vi "ReCalc_V2.00.vi"(3 "Berechnen":bool, 4 "Datenspeicher":T2={"Fahrzeugdaten"="", "date/time string"="", "Rolle [Inkr/U]"=0, "Rollenumfang [m]"=0.0, "Rollenträgheit [kgm²]"=0.0, "Zündung [Imp/U]"=0.0, "Getriebe [1:]"=0.0, "Reifenumfang [m] "=0.0, "element"=0.0, "Gl. Mittelwert"=0, "Differenzenquotient"=0, "Polynom"=0, "dT [s]"=0.0, "element"=0.0, "Lufttemperatur [°C]"=0.0, "Luftfeuchtigkeit [%]"=0.0, "Luftdruck [mbar]"=0.0, [], [], "Best Polynomial Fit"=[], [], "Übersetzung ermitteln aus"=0, "[s]"=0.0, "nmin [1/min]"=0.0, "nmax [1/min]"=0.0, "n vom Gas [1/min]"=0.0, "dT ungefiltert [s]"=[], [], "Boolesch"=FALSE, "Serielle Schnittstelle"="COM4", "nKuWe/nRolle 2"=10.0}) -> ()   [LabVIEW 2014]
uses:
  <vilib>/Utility/miscctls.llb/LVPointTypeDef.ctl
  <vilib>/Utility/xml.llb/Read From XML File(string).vi
  <vilib>/Analysis/3filter.llb/IIR Filter (DBL).vi
  <vilib>/Analysis/NI_AALBase.lvlib
panel:
  in  "Legende":bool=TRUE
  out "Fahrzeugdaten":string
  out "Überlagerung":bool
  in  "Überlagern":bool
  out "Übersetzung ermitteln aus":T1(ring)
  in  "Speichern":bool
  out "Reifenumfang [m]":dbl=1.222
  out "Getriebe [1:]":dbl=5.343
  out "Zündung [Imp/U]":dbl=1.0
  out "Rollengeber [Inkr/U]":u16=200
  out "Luftdruck [mbar]":dbl=1013.0
  out "Luftfeuchtigkeit [%]":dbl=50.0
  out "Lufttemperatur [°C]":dbl=20.0
  in  "Stopp":bool
  in  "Rollenträgheit [kgm²]":dbl=0.402
  in  "Gl. Mittelwert":u8=35
  in  "Differenzenquotient":u8=12
  in  "n vom Gas [1/min]":dbl=5000.0
  out "Rollenumfang [m]":dbl=0.613 format="%.3f"
  out "Datum, Zeit":string
  out "Untersetzung aus:":dbl=2.68 format="%.2f"
  in  "Drucken":bool
  out "Pmax":string
  out "Ergebnis":string
  out "XY-Graph":cluster{dbl[], dbl[]}[](graph)
  in  "Öffnen":bool
  out "korr":dbl
  out "[s]":dbl=5.0
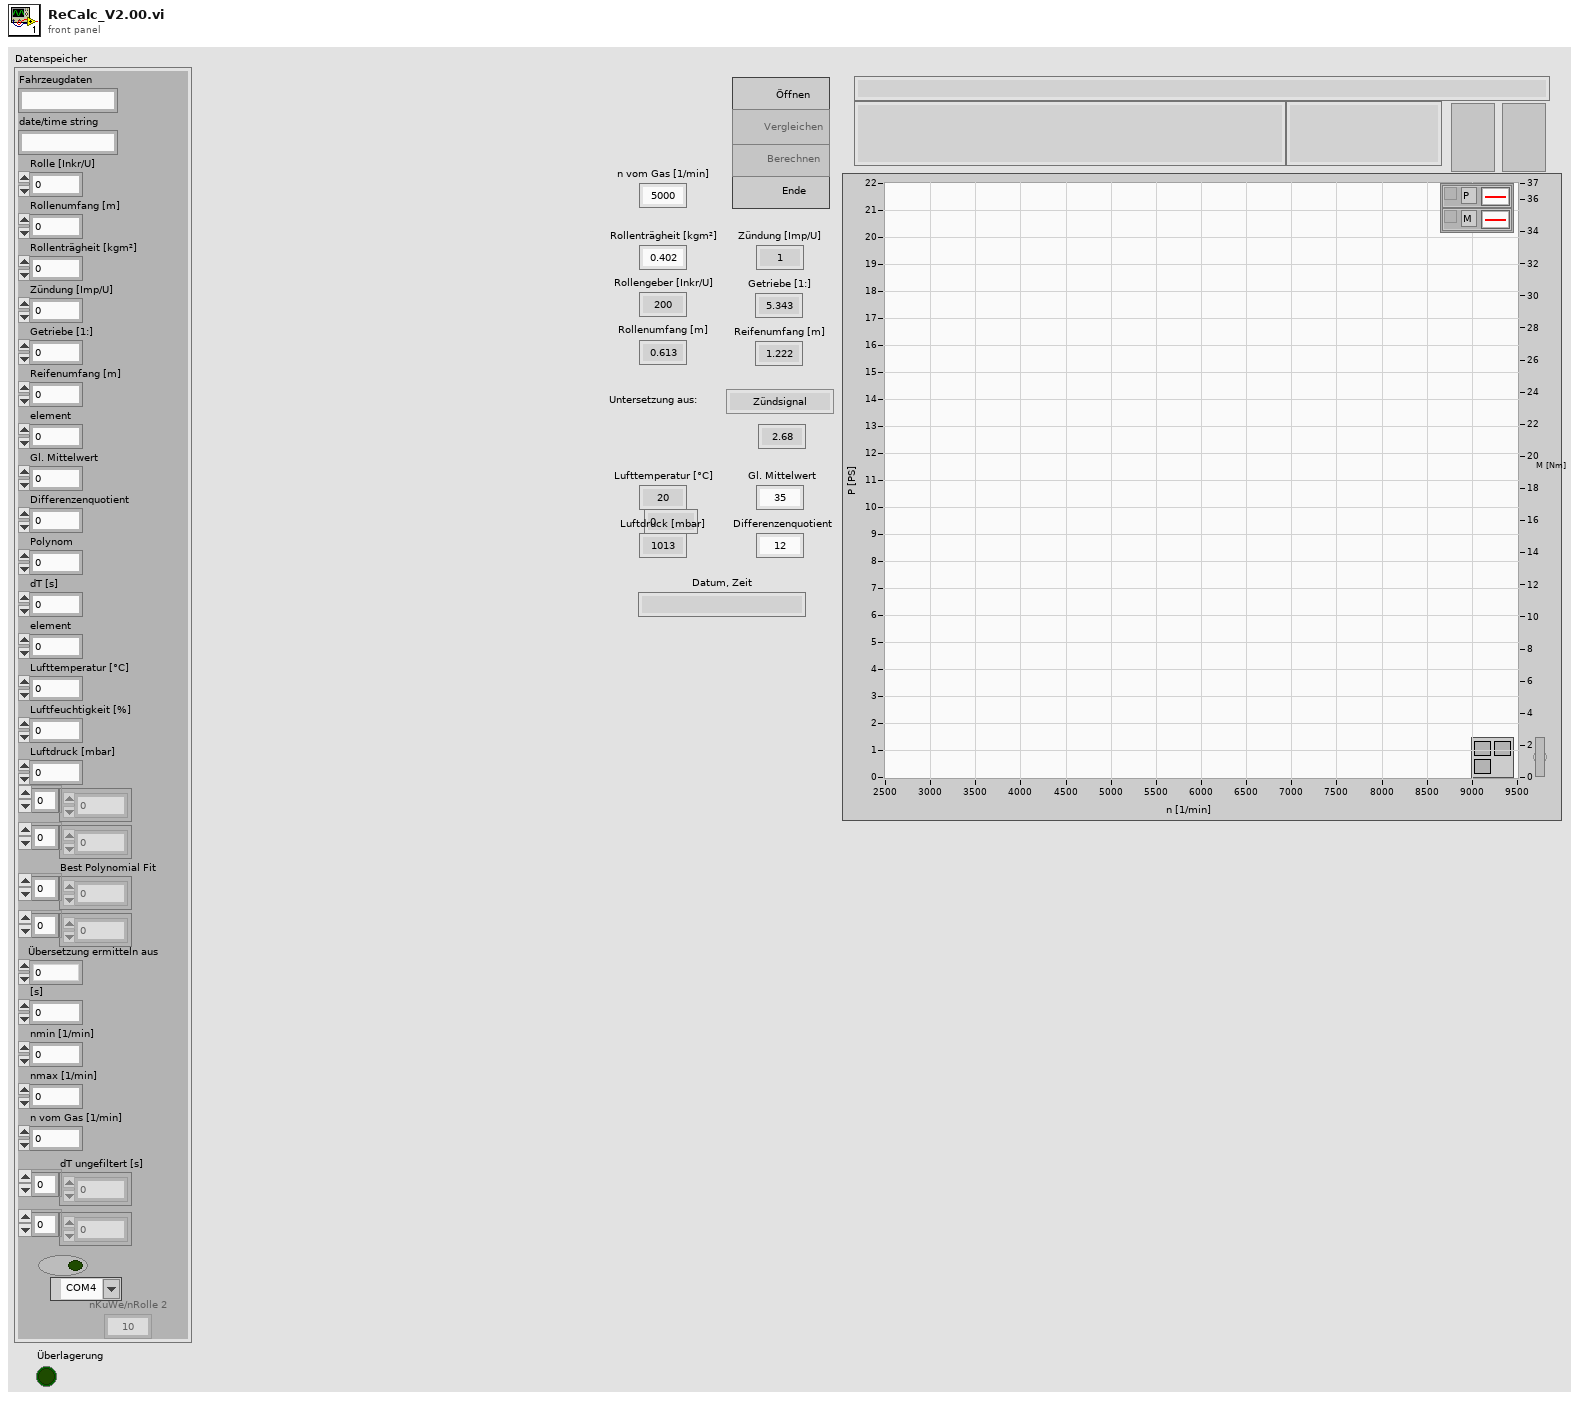
[diagram p1: front panel]
types:
  T1 = enum8{"Zündsignal", "Getriebe & Reifen", "nKuWe / nRolle :"}
  T2 = cluster{"Fahrzeugdaten":string, "date/time string":string, "Rolle [Inkr/U]":u16, "Rollenumfang [m]":dbl, "Rollenträgheit [kgm²]":dbl, "Zündung [Imp/U]":dbl, "Getriebe [1:]":dbl, "Reifenumfang [m] ":dbl, "element":dbl, "Gl. Mittelwert":u8, "Differenzenquotient":u8, "Polynom":u8, "dT [s]":dbl, "element":dbl, "Lufttemperatur [°C]":dbl, "Luftfeuchtigkeit [%]":dbl, "Luftdruck [mbar]":dbl, dbl[], dbl[], "Best Polynomial Fit":dbl[], dbl[], "Übersetzung ermitteln aus":u8, "[s]":dbl, "nmin [1/min]":dbl, "nmax [1/min]":dbl, "n vom Gas [1/min]":dbl, "dT ungefiltert [s]":dbl[], i32[], "Boolesch":bool, "Serielle Schnittstelle":refnum<visa-resource-name>, "nKuWe/nRolle 2":dbl}
  T3 = typedef "LVPointTypeDef.ctl" = cluster{"Horizontal":i16, "Vertical":i16}
  T4 = enum8{"Enabled", "Disabled", "Disabled and Grayed Out"}
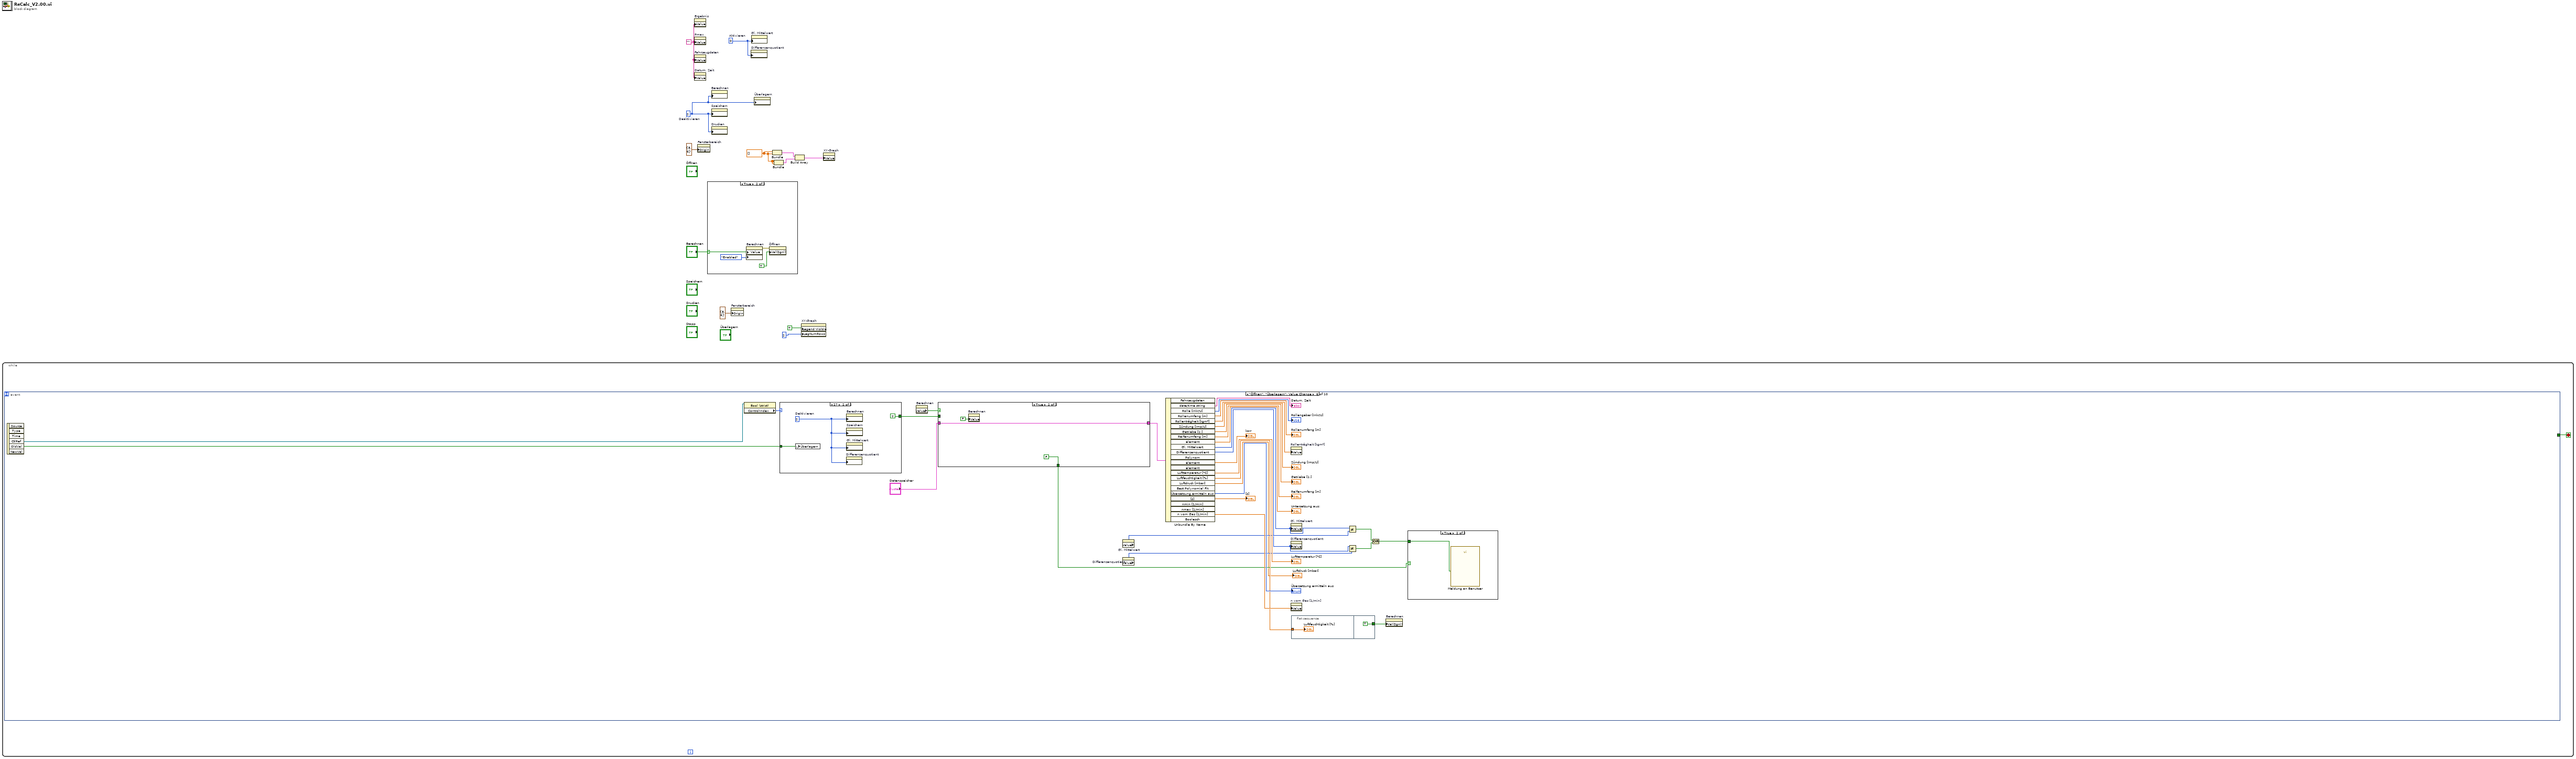
[diagram p0: block diagram]
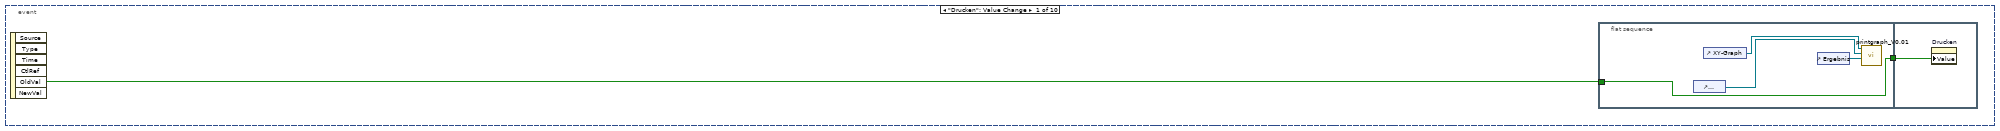
[diagram p3: hidden frame]
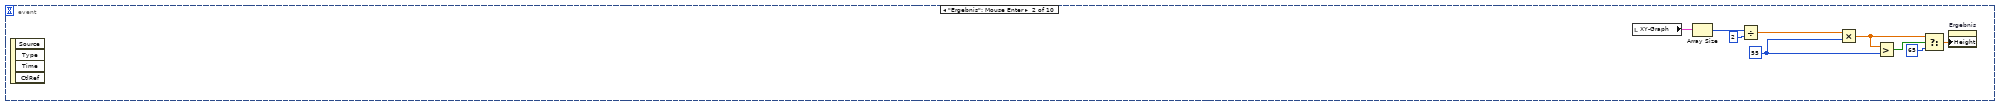
[diagram p4: hidden frame]
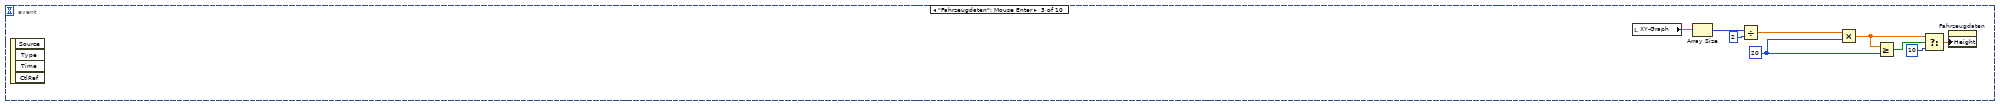
[diagram p5: hidden frame]
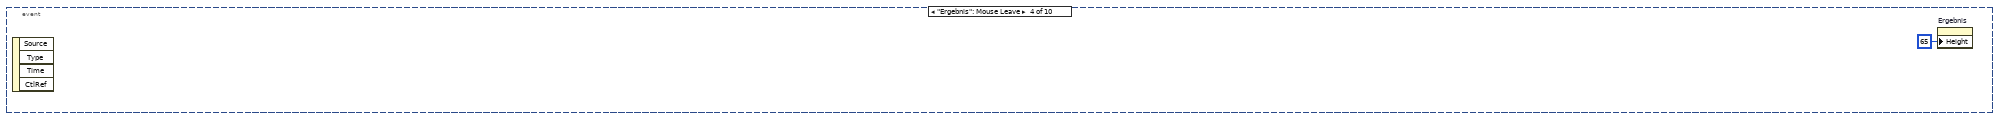
[diagram p6: hidden frame]
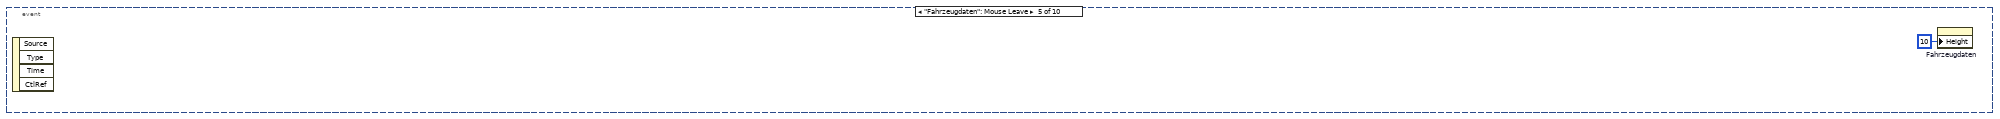
[diagram p7: hidden frame]
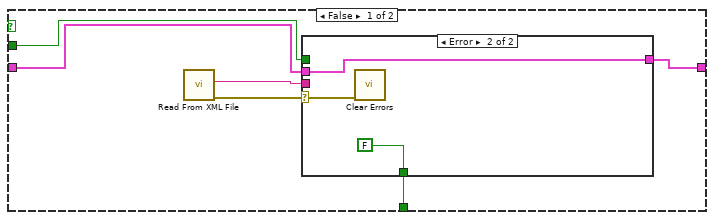
[diagram p9: hidden frame]
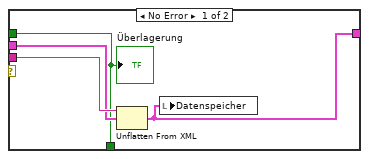
[diagram p10: hidden frame]
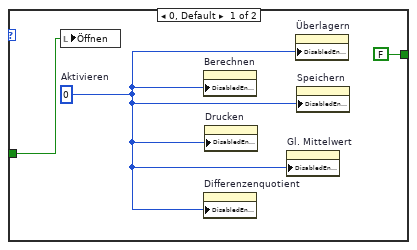
[diagram p11: hidden frame]
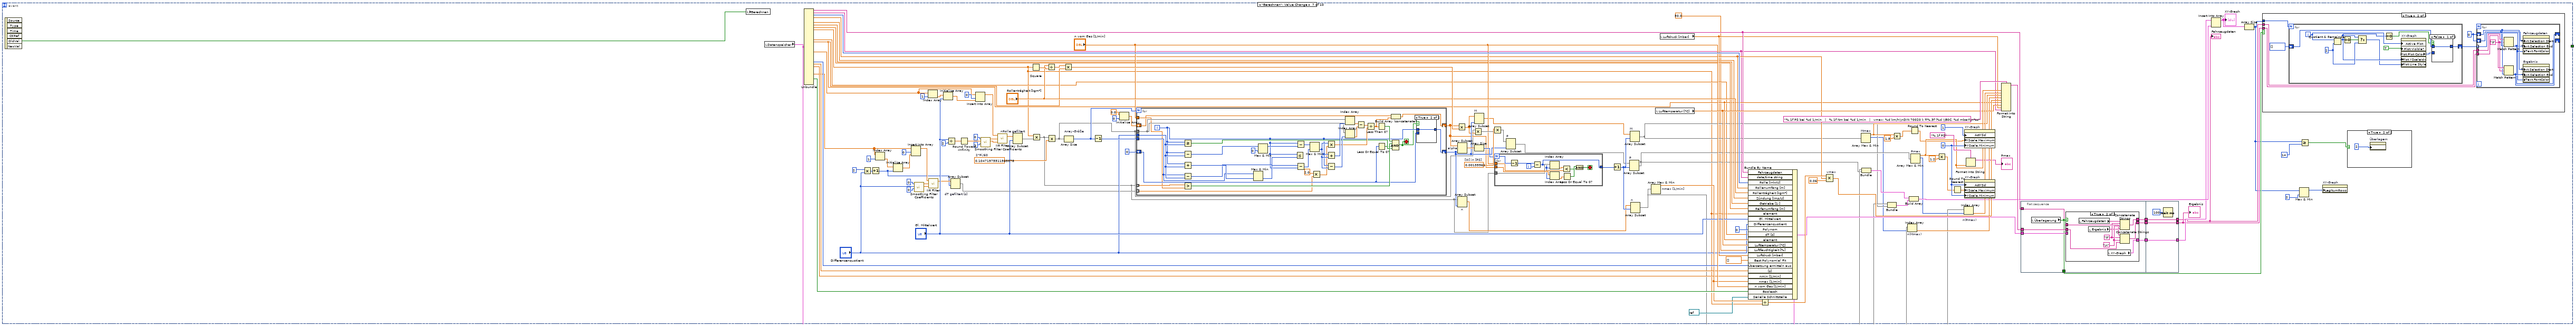
[diagram p12: hidden frame]
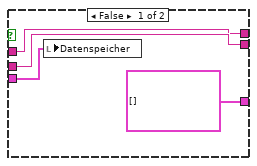
[diagram p14: hidden frame]
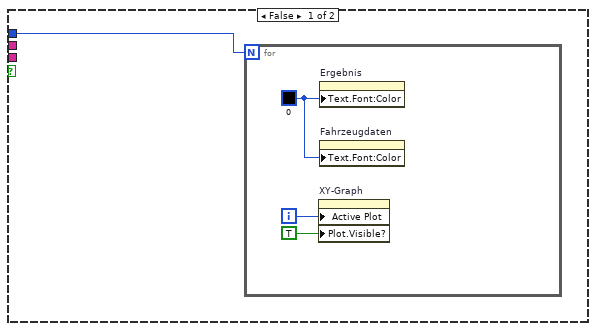
[diagram p15: hidden frame]
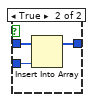
[diagram p16: hidden frame]
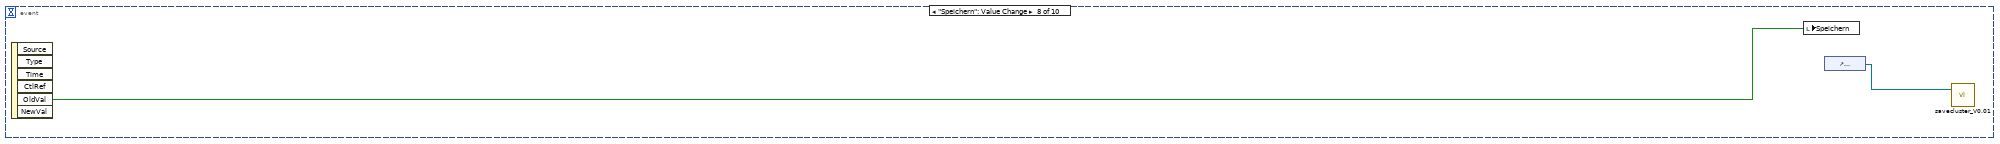
[diagram p18: hidden frame]
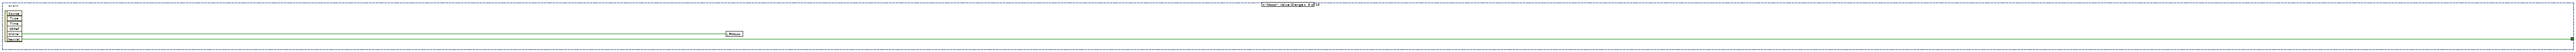
[diagram p19: hidden frame]
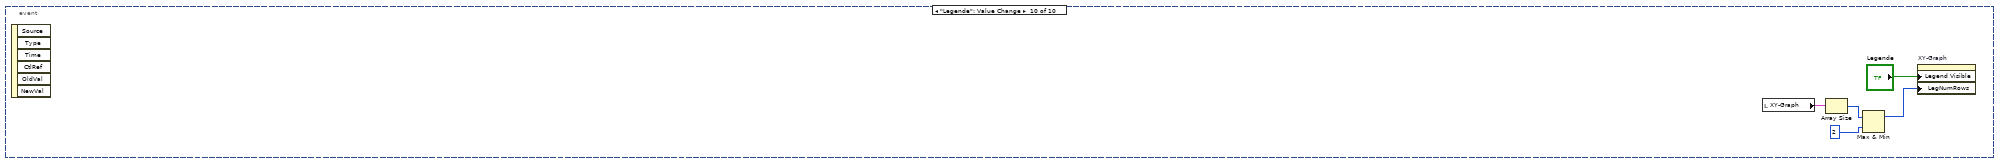
[diagram p20: hidden frame]
diagram:
  w2 = 0  # Aktivieren
  w8 = dbl[] []
  w4 = 2  # Deaktivieren
  w12 = ""
  n1 = while {
    stop <- w13 stop-if-true
    n2 = event shown="[5] \"Öffnen\", \"Überlagern\": Value Change" {
      selector: _ -> [_ _ _ _ _ _ _ _ _ _]
      dyn-events: _ -> [_ _ _ _ _ _ _ _ _ _]
      timeout: _ -> [_ _ _ _ _ _ _ _ _ _]
      tunnel: [_ _ _ _ _ _ _ _ w328 _] -> w13
      event "Drucken": Value Change {
        n3 = event-data() -> ("OldVal"=w15:bool)  [unwired: 1 in, 5 out]
        n4 = flat-sequence {
          tunnel: w15 -> [w19]
          tunnel: [w19] -> w14
          tunnel: w14 -> [w20]
          frame #0 {
            n5 = control-ref of="Fahrzeugdaten"() -> (w17:refnum<vi>)
            n6 = control-ref of="XY-Graph"() -> (w18:refnum<vi>)
            n7 = control-ref of="Ergebnis"() -> (w16:refnum<vi>)
            n8 = call "printgraph_V0.01.vi"("reference 2"=w16, "Fahrzeugdaten"=w17, "XYGraph (Eingang)"=w18) -> ()  [unwired: 9 in]
          }
          frame #1 {
            n9 = property on="Drucken" class="Bool. (strikt)"("Value"=w20) -> ()  [unwired: 2 in, 2 out]
          }
        }
      }
      event "Ergebnis": Mouse Enter {
        w23 = u32 55 ("Größe:Höhe")
        n10 = event-data() -> ()  [unwired: 1 in, 4 out]
        n11 = local read "XY-Graph"() -> (w29:cluster{dbl[], dbl[]}[])
        n12 = Array Size(array=w29) -> (size(s)=w28:i32)
        n13 = Divide(x=w28, y=2) -> (x/y=w26:dbl)
        n14 = Multiply(x=w26, y=w23) -> (x*y=w24:dbl)
        n15 = Greater?(x=w24, y=w23) -> (0:w25:bool)
        n16 = Select(t=w24, s=w25, f=u32 65 ("Größe:Höhe")) -> (s? t:f=w22:dbl)
        n17 = property on="Ergebnis" class="Str"("Height"=w22) -> ()  [unwired: 2 in, 2 out]
      }
      event "Fahrzeugdaten": Mouse Enter {
        w32 = u32 20 ("Größe:Höhe")
        n18 = event-data() -> ()  [unwired: 1 in, 4 out]
        n19 = local read "XY-Graph"() -> (w38:cluster{dbl[], dbl[]}[])
        n20 = Array Size(array=w38) -> (size(s)=w37:i32)
        n21 = Divide(x=w37, y=2) -> (x/y=w35:dbl)
        n22 = Multiply(x=w35, y=w32) -> (x*y=w33:dbl)
        n23 = Greater Or Equal?(x=w33, y=w32) -> (x >= y?=w34:bool)
        n24 = Select(t=w33, s=w34, f=u32 10 ("Größe:Höhe")) -> (s? t:f=w31:dbl)
        n25 = property on="Fahrzeugdaten" class="Str"("Height"=w31) -> ()  [unwired: 2 in, 2 out]
      }
      event "Ergebnis": Mouse Leave {
        n26 = event-data() -> ()  [unwired: 1 in, 4 out]
        n27 = property on="Ergebnis" class="Str"("Height"=u32 65 ("Größe:Höhe")) -> ()  [unwired: 2 in, 2 out]
      }
      event "Fahrzeugdaten": Mouse Leave {
        n28 = event-data() -> ()  [unwired: 1 in, 4 out]
        n29 = property on="Fahrzeugdaten" class="Str"("Height"=u32 10 ("Größe:Höhe")) -> ()  [unwired: 2 in, 2 out]
      }
      event "Öffnen", "Überlagern": Value Change {
        n30 = event-data() -> ("CtlRef"=w70:refnum<vi>, "OldVal"=w68:bool)  [unwired: 1 in, 4 out]
        n31 = property class="Bool (strict)"(reference=w70) -> ("ControlIndex"=w69:i32)  [unwired: 1 in, 2 out]
        n32 = case shown="27" w69 {
          tunnel: w68 -> [w93 w96]
          tunnel: [FALSE ("Überlagerung") TRUE ("Überlagerung")] -> w67
          frame 0, Default {
            w91 = 0  # Aktivieren
            n33 = local write "Öffnen"(w93) -> ()
            n34 = property on="Berechnen" class="Bool. (strikt)"("DisabledEnum"=w91) -> ()  [unwired: 2 in, 2 out]
            n35 = property on="Differenzenquotient" class="DigWert (strikt)"("DisabledEnum"=w91) -> ()  [unwired: 2 in, 2 out]
            n36 = property on="Drucken" class="Bool. (strikt)"("DisabledEnum"=w91) -> ()  [unwired: 2 in, 2 out]
            n37 = property on="Gl. Mittelwert" class="DigWert (strikt)"("DisabledEnum"=w91) -> ()  [unwired: 2 in, 2 out]
            n38 = property on="Überlagern" class="Bool. (strikt)"("DisabledEnum"=w91) -> ()  [unwired: 2 in, 2 out]
            n39 = property on="Speichern" class="Bool. (strikt)"("DisabledEnum"=w91) -> ()  [unwired: 2 in, 2 out]
          }
          frame 27 {
            w94 = 2  # Dektivieren
            n40 = local write "Überlagern"(w96) -> ()
            n41 = property on="Differenzenquotient" class="DigWert (strikt)"("DisabledEnum"=w94) -> ()  [unwired: 2 in, 2 out]
            n42 = property on="Berechnen" class="Bool. (strikt)"("DisabledEnum"=w94) -> ()  [unwired: 2 in, 2 out]
            n43 = property on="Speichern" class="Bool. (strikt)"("DisabledEnum"=w94) -> ()  [unwired: 2 in, 2 out]
            n44 = property on="Gl. Mittelwert" class="DigWert (strikt)"("DisabledEnum"=w94) -> ()  [unwired: 2 in, 2 out]
          }
        }
        n45 = property on="Berechnen" class="Bool. (strikt)"() -> ("Value"=w50:bool)  [unwired: 2 in, 2 out]
        n46 = case shown="True" w50 {
          tunnel: "Datenspeicher" -> [w77 w87]
          tunnel: w67 -> [w75 _]
          tunnel: [w74 w87] -> w51
          tunnel: [w73 FALSE] -> w45
          frame False {
            n47 = call-poly <vilib>:"Read From XML File.vi"() -> ("error out"=w76:errorcluster, "XML Elements"=w78:string)  [unwired: 9 in, 1 out]
            n48 = case shown="Error" w76 {
              selector: w76 -> [_ w85]
              tunnel: w78 -> [w82 _]
              tunnel: w77 -> [w81 w84]
              tunnel: w75 -> [w79 _]
              tunnel: [w80 w84] -> w74
              tunnel: [w79 FALSE] -> w73
              frame No Error {
                n49 = Unflatten From XML(xml string=w82, type=w81) -> (value=w80:T2)  [unwired: 1 in, 1 out]
                n50 = local write "Datenspeicher"(w80) -> ()
                "Überlagerung" <- w79
              }
              frame Error {
                n51 = call <vilib>:"Clear Errors.vi"("error in (no error)"=w85) -> ()  [unwired: 5 in, 2 out]
              }
            }
          }
          frame True {
            n52 = property on="Berechnen" class="Bool. (strikt)"("Value"=FALSE) -> ()  [unwired: 2 in, 2 out]
          }
        }
        n53 = property on="Gl. Mittelwert" class="DigWert (strikt)"() -> ("Value"=w48:u8)  [unwired: 2 in, 2 out]
        n54 = property on="Differenzenquotient" class="DigWert (strikt)"() -> ("Value"=w46:u8)  [unwired: 2 in, 2 out]
        n55 = Unbundle By Name(w51) -> ("date/time string"=→"Datum, Zeit":string, "Rolle [Inkr/U]"=→"Rollengeber [Inkr/U]":u16, "Rollenumfang [m]"=→"Rollenumfang [m]":dbl, "Rollenträgheit [kgm²]"=w56:dbl, "Zündung [Imp/U]"=→"Zündung [Imp/U]":dbl, "Getriebe [1:]"=→"Getriebe [1:]":dbl, "Reifenumfang [m]"=→"Reifenumfang [m]":dbl, "element"=→"Untersetzung aus:":dbl, "Gl. Mittelwert"=w49:u8, "Differenzenquotient"=w47:u8, "element"=→"korr":dbl, "Lufttemperatur [°C]"=→"Lufttemperatur [°C]":dbl, "Luftfeuchtigkeit [%]"=w63:dbl, "Luftdruck [mbar]"=→"Luftdruck [mbar]":dbl, "Übersetzung ermitteln aus"=→"Übersetzung ermitteln aus":u8, "[s]"=→"[s]":dbl, "n vom Gas [1/min]"=w66:dbl)  [unwired: 7 out]
        n56 = property on="Rollenträgheit [kgm²]" class="DigWert (strikt)"("Value"=w56) -> ()  [unwired: 2 in, 2 out]
        n57 = property on="Gl. Mittelwert" class="DigWert (strikt)"("Value"=w49) -> ()  [unwired: 2 in, 2 out]
        n58 = property on="Differenzenquotient" class="DigWert (strikt)"("Value"=w47) -> ()  [unwired: 2 in, 2 out]
        n59 = property on="n vom Gas [1/min]" class="DigWert (strikt)"("Value"=w66) -> ()  [unwired: 2 in, 2 out]
        n60 = flat-sequence {
          tunnel: w63 -> [w89]
          tunnel: [TRUE] -> w52
          frame #0 {
            "Luftfeuchtigkeit [%]" <- w89
          }
          frame #1 {
          }
        }
        n61 = Not Equal?(x=w49, y=w48) -> (x != y?=w44:bool)
        n62 = Not Equal?(x=w47, y=w46) -> (x != y?=w43:bool)
        n63 = Or(x=w44, y=w43) -> (x .or. y?=w42:bool)
        n64 = property on="Berechnen" class="Bool. (strikt)"("Val(Sgnl)"=w52) -> ()  [unwired: 2 in, 2 out]
        n65 = case shown="True" w45 {
          tunnel: w42 -> [_ w72]
          frame False {
          }
          frame True {
            n66 = call "Meldung an Benutzer"("Enable"=w72) -> ()  [unwired: 9 in, 2 out]
          }
        }
      }
      event "Berechnen": Value Change {
        w193 = 0
        w207 = 0.00135962  # [W] in [PS]
        w214 = 0.10471975511965978  # 2*Pi/60
        n67 = event-data() -> ("OldVal"=w155:bool)  [unwired: 1 in, 5 out]
        n68 = local write "Berechnen"(w155) -> ()
        n69 = local read "Datenspeicher"() -> (w173:T2)
        n70 = Unbundle(w173) -> ("Fahrzeugdaten"=w147:string, "date/time string"=w98:string, "Rolle [Inkr/U]"=w171:u16, "Rollenumfang [m]"=w164:dbl, "Zündung [Imp/U]"=w163:dbl, "Getriebe [1:]"=w162:dbl, "Reifenumfang [m]"=w161:dbl, "element"=w107:dbl, "dT [s]"=w117:dbl, "element"=w160:dbl, w116:dbl[], "Übersetzung ermitteln aus"=w165:u8, "[s]"=w157:dbl, "nmin [1/min]"=w158:dbl, "dT ungefiltert [s]"=w115:dbl[], "Boolesch"=w168:bool)  [unwired: 15 out]
        n71 = Multiply(x=2, y="Differenzenquotient") -> (x*y=w125:i32)
        n72 = Increment(x=w125) -> (x+1=w118:i32)
        n73 = Index Array(array=w115, index=1 ("Index")) -> (element=w123:dbl)
        n74 = Initialize Array(w123, w118) -> (w121:dbl[])
        n75 = Insert Into Array(array=w115, index=0 ("Index"), new element=w121) -> (w120:dbl[])
        n76 = call <vilib>:"Smoothing Filter Coefficients.vi"("shape"=0, "half-width"="Differenzenquotient", "type"=0) -> ("forward coefficients"=w128:dbl[], "reverse coefficients"=w129:dbl[])  [unwired: 6 in, 1 out]
        n77 = Index Array(array=w116, index=1) -> (element=w178:dbl)
        n78 = call-poly <vilib>:"IIR Filter.vi"("Forward Coefficients"=w128, "Reverse Coefficients"=w129, "X"=w120) -> ("Filtered X"=w119:dbl[])  [unwired: 1 in, 1 out]
        n79 = Initialize Array(w178, "Gl. Mittelwert") -> (w179:dbl[])
        n80 = Divide(x="Gl. Mittelwert", y=2) -> (x/y=w217:dbl)
        n81 = Array Subset "dT gefiltert [s]"(array=w119, index=w118) -> (w110:dbl[])  [unwired: 1 in]
        n82 = Round Toward -Infinity(1:w217) -> (0:w216:dbl)
        n83 = Insert Into Array ("In Array einfügen")(array=w116, index=0, new element=w179) -> (w176:dbl[])
        n84 = call <vilib>:"Smoothing Filter Coefficients.vi"("shape"=1, "half-width"=w216, "type"=0) -> ("forward coefficients"=w180:dbl[], "reverse coefficients"=w181:dbl[])  [unwired: 6 in, 1 out]
        n85 = call-poly <vilib>:"IIR Filter.vi"("Forward Coefficients"=w180, "Reverse Coefficients"=w181, "X"=w176) -> ("Filtered X"=w175:dbl[])  [unwired: 1 in, 1 out]
        n86 = Array Subset "nRolle gefiltert"(array=w175, index="Gl. Mittelwert") -> (w109:dbl[])  [unwired: 1 in]
        n87 = Square(x=w107) -> (x^2=w208:dbl)
        n88 = Multiply(x=w107, y=w109) -> (x*y=w108:dbl[])
        n89 = Divide(x="Rollenträgheit [kgm²]", y=w208) -> (x/y=w205:dbl)
        n90 = Multiply(x=w108, y=w214) -> (x*y=w111:dbl[])
        n91 = Multiply(x=w205, y=w160) -> (x*y=w204:dbl)
        n92 = Array Size "Array-Größe"(array=w111) -> (size(s)=w212:i32)
        n93 = Decrement(x=w212) -> (x-1=w213:i32)
        n94 = Initialize Array(0.0 ("y"), 0) -> (w209:dbl[])
        n95 = for {
          N: w212 -> [_]
          tunnel: "Differenzenquotient" -> [w303]
          tunnel: w111 -> [w309]
          tunnel: w213 -> [w302]
          shift-right: [w307] -> w112
          shift-left: w209 -> [w290]
          tunnel: w108 -> [w305] mode=indexing
          tunnel: "n vom Gas [1/min]" -> [w294]
          shift-right: [w293] -> w200
          shift-left: 0 -> [w296]
          tunnel: w110 -> [w289] mode=indexing
          i -> [w297]
          stop <- w295 stop-if-true
          n96 = Greater Or Equal?(x=w297, y=w303) -> (x >= y?=w300:bool)
          n97 = Subtract(x=w297, y=w303) -> (x-y=w322:i32)
          n98 = Add(x=w297, y=w303) -> (x+y=w316:i32)
          n99 = Subtract(x=w302, y=w303) -> (x-y=w304:i32)
          n100 = Greater?(x=w305, y=w294) -> (0:w306:bool)
          n101 = Max & Min(x=w302, y=w316) -> (min(x,y)=w317:i32)  [unwired: 1 out]
          n102 = Max & Min(x=w322, y=0) -> (max(x,y)=w320:i32)  [unwired: 1 out]
          n103 = Less Or Equal?(x=w297, y=w304) -> ()  [unwired: 1 out]
          n104 = Subtract(x=w297, y=w320) -> (x-y=w319:i32)
          n105 = Subtract(x=w317, y=w297) -> (x-y=w318:i32)
          n106 = Max & Min(x=w319, y=w318) -> (min(x,y)=w310:i32)  [unwired: 1 out]
          n107 = Multiply(x=2.0, y=w289) -> (x*y=w291:dbl)
          n108 = Multiply(x=w310, y=w291) -> (x*y=w308:dbl)
          n109 = Add(x=w297, y=w310) -> (x+y=w315:i32)
          n110 = Subtract(x=w297, y=w310) -> (x-y=w314:i32)
          n111 = Index Array(array=w309, index=w315) -> (element=w312:dbl)
          n112 = Index Array(array=w309, index=w314) -> (element=w313:dbl)
          n113 = Subtract(x=w312, y=w313) -> (x-y=w311:dbl)
          n114 = Divide(x=w311, y=w308) -> (x/y=w301:dbl)
          n115 = Less Than 0?(x=w301) -> (x < 0?=w299:bool)
          n116 = Less Or Equal To 0?(x=w296) -> (x <= 0?=w298:bool)
          n117 = Build Array (concatenate)(w290, w301) -> (w307:dbl[])
          n118 = Compound Arithmetic op=AND(w299, w306, w298, w300) -> (w295:bool)
          n119 = case shown="True" w295 {
            tunnel: w297 -> [_ w324]
            tunnel: [w323 w324] -> w293
            tunnel: w296 -> [w323 _]
            frame False {
            }
            frame True {
            }
          }
        }
        n120 = Multiply(x=w112, y=w204) -> (x*y=w184:dbl[])
        n121 = Array Subset "alpha"(array=w112, length=w200) -> (w202:dbl[])  [unwired: 1 in]
        n122 = Array Subset "n"(array=w108, length=w200) -> (w182:dbl[])  [unwired: 1 in]
        n123 = Multiply(x=w111, y=w184) -> (x*y=w206:dbl[])
        n124 = Array Subset "M"(array=w184, length=w200) -> (w114:dbl[])  [unwired: 1 in]
        n125 = Array Size(array=w202) -> (size(s)=w199:i32)
        n126 = Multiply(x=w207, y=w206) -> (x*y=w201:dbl[])
        n127 = for {
          N: w199 -> [w288]
          tunnel: w112 -> [w285]
          tunnel: w108 -> [w282]
          tunnel: "n vom Gas [1/min]" -> [w279]
          tunnel: [w277] -> w198
          i -> [w283]
          stop <- w278 stop-if-true
          n128 = Decrement(x=w288) -> (x-1=w287:i32)
          n129 = Subtract(x=w287, y=w283) -> (x-y=w277:i32)
          n130 = Index Array(array=w282, index=w277) -> (element=w281:dbl)
          n131 = Index Array(array=w285, index=w277) -> (element=w286:dbl)
          n132 = Less?(x=w281, y=w279) -> (x < y?=w280:bool)
          n133 = Less Or Equal To 0?(x=w286) -> (x <= 0?=w284:bool)
          n134 = And(x=w284, y=w280) -> (x .and. y?=w278:bool)
        }
        n135 = Array Subset "P"(array=w201, length=w200) -> (w113:dbl[])  [unwired: 1 in]
        n136 = Increment(x=w198) -> (x+1=w197:i32)
        n137 = Array Subset "P"(array=w113, index=w197) -> (w138:dbl[])  [unwired: 1 in]
        n138 = Array Subset "M"(array=w114, index=w197) -> (w136:dbl[])  [unwired: 1 in]
        n139 = Array Subset "n"(array=w182, index=w197) -> (w140:dbl[])  [unwired: 1 in]
        n140 = Array Max & Min "nmax [1/min]"(array=w140) -> (max value=w159:dbl)  [unwired: 3 out]
        n141 = local read "Lufttemperatur [°C]"() -> (w172:dbl)
        n142 = local read "Luftdruck [mbar]"() -> (w99:dbl)
        n143 = Bundle By Name(cluster=w173, "Fahrzeugdaten"=w147, "date/time string"=w98, "Rolle [Inkr/U]"=w171, "Rollenumfang [m]"=w164, "Rollenträgheit [kgm²]"="Rollenträgheit [kgm²]", "Zündung [Imp/U]"=w163, "Getriebe [1:]"=w162, "Reifenumfang [m]"=w161, "element"=w107, "Gl. Mittelwert"="Gl. Mittelwert", "Differenzenquotient"="Differenzenquotient", "Polynom"=0, "dT [s]"=w117, "element"=w160, "Lufttemperatur [°C]"=w172, "Luftfeuchtigkeit [%]"=50.0, "Luftdruck [mbar]"=w99, "Best Polynomial Fit"=dbl[] [], "Übersetzung ermitteln aus"=w165, "[s]"=w157, "nmin [1/min]"=w158, "nmax [1/min]"=w159, "n vom Gas [1/min]"="n vom Gas [1/min]", "Boolesch"=w168, "Serielle Schnittstelle"=refnum<visa-resource-name> refnum) -> (w153:T2)
        n144 = Divide(x=w159, y=w107) -> (x/y=w192:dbl)
        n145 = Compound Arithmetic op=MULTIPLY "vmax"(w192, w164, 0.06) -> (w189:dbl)
        n146 = Array Max & Min "Mmax"(array=w136) -> (max value=w186:dbl, max index (indices)=w135:i32)  [unwired: 2 out]
        n147 = Bundle(w140, w138) -> (w142:cluster{dbl[], dbl[]})  [unwired: 1 in]
        n148 = Bundle(w140, w136) -> (w141:cluster{dbl[], dbl[]})  [unwired: 1 in]
        n149 = Multiply(x=w186, y=1.8) -> (x*y=w106:dbl)
        n150 = Index Array "n(Mmax)"(array=w140, index=w135) -> (element=w166:dbl)
        n151 = Build Array(w142, w141) -> (w151:cluster{dbl[], dbl[]}[])
        n152 = Round To Nearest(number=w106) -> (nearest integer value=w105:dbl)
        n153 = Array Max & Min "Pmax"(array=w138) -> (max value=w187:dbl, max index (indices)=w134:i32)  [unwired: 2 out]
        n154 = Multiply(x=w187, y=1.2) -> (x*y=w103:dbl)
        n155 = Round To Nearest(number=w103) -> (nearest integer value=w104:dbl)
        n156 = Index Array "n(Pmax)"(array=w140, index=w134) -> (element=w190:dbl)
        n157 = property on="XY-Graph" class="XYGraph (strikt)"("ActYScl"=1, "YScale.Maximum"=w105, "YScale.Minimum"=w193) -> ()  [unwired: 2 in, 2 out]
        n158 = property on="XY-Graph" class="XYGraph (strikt)"("ActYScl"=w193, "YScale.Maximum"=w104, "YScale.Minimum"=w193) -> ()  [unwired: 2 in, 2 out]
        n159 = Format Into String(format string="%.1f PS" ("Format-String"), w187) -> (resulting string=→"Pmax":string)  [unwired: 2 in, 1 out]
        n160 = Format Into String(format string="%.1f PS bei %d 1/min   |   %.1f Nm bei %d 1/min   |   vmax: %d km/h\\nDIN 70020 k =%.3f (%d \\B0C, %d mbar)\\n%s" ("Format-String"), w187, w190, w186, w166, w189, w160, w172, w99, w98) -> (resulting string=w156:string)  [unwired: 2 in, 1 out]
        n161 = flat-sequence {
          tunnel: w156 -> [w227]
          tunnel: w153 -> [w226]
          tunnel: [w225] -> w152
          tunnel: w147 -> [w221]
          tunnel: [w224] -> w146
          tunnel: [w223] -> w145
          tunnel: [w222] -> w144
          tunnel: [w242] -> w148
          tunnel: [w243] -> w149
          tunnel: [w244] -> w150
          tunnel: w146 -> [w244]
          tunnel: w145 -> [w243]
          tunnel: w144 -> [w242]
          frame #0 {
            n162 = local read "Überlagerung"() -> (w225:bool)
            n163 = case shown="True" w225 {
              tunnel: [cluster{dbl[], dbl[]}[] [] ("XY-Graph") w240] -> w224
              tunnel: w227 -> [w230 w238]
              tunnel: [w230 w239] -> w223
              tunnel: w226 -> [w229 _]
              tunnel: w221 -> [w228 w236]
              tunnel: [w228 w235] -> w222
              frame False {
                n164 = local write "Datenspeicher"(w229) -> ()
              }
              frame True {
                w234 = "\t"
                w237 = "\n"
                n165 = local read "Fahrzeugdaten"() -> (w233:string)
                n166 = local read "Ergebnis"() -> (w232:string)
                n167 = local read "XY-Graph"() -> (w240:cluster{dbl[], dbl[]}[])
                n168 = Concatenate Strings(w233, w234, w237, w236) -> (w235:string)
                n169 = Concatenate Strings(w232, w234, w237, w238) -> (w239:string)
              }
            }
          }
          frame #1 {
            n170 = Wait (ms)(milliseconds to wait=u32 100 ("Zu wartende ms")) -> ()  [unwired: 1 out]
          }
        }
        n171 = Insert Into Array(array=w150, new element=w151) -> (w154:cluster{dbl[], dbl[]}[])  [unwired: 1 in]
        "XY-Graph" <- w154
        n172 = Array Size(array=w154) -> (size(s)=w100:i32)
        n173 = case shown="True" w152 {
          tunnel: w100 -> [w245 w254]
          tunnel: w149 -> [_ w251]
          tunnel: w148 -> [_ w250]
          frame False {
            n174 = for {
              N: w245 -> [_]
              i -> [w248]
              w246 = u32 0
              n175 = property on="XY-Graph" class="XYGraph (strikt)"("Active Plot"=w248, "Plot.Visible?"=TRUE ("Plot.Sichtbar")) -> ()  [unwired: 2 in, 2 out]
              n176 = property on="Ergebnis" class="Str"("Text.Font:Color"=w246) -> ()  [unwired: 2 in, 2 out]
              n177 = property on="Fahrzeugdaten" class="Str"("Text.Font:Color"=w246) -> ()  [unwired: 2 in, 2 out]
            }
          }
          frame True {
            w249 = 0
            n178 = for {
              N: w254 -> [_]
              shift-right: [w272] -> w252
              shift-left: u32[] [] -> [w271]
              i -> [w266]
              w269 = 2 ("y")
              n179 = Quotient & Remainder(x=w266, y=w269) -> (x-y*floor(x/y)=w264:i32)  [unwired: 1 out]
              n180 = Equal To 0?(x=w264) -> (x = 0?=w268:bool)
              n181 = Select(t=w264, s=w268, f=w269) -> (s? t:f=w263:i32)
              n182 = Equal To 0?(x=w264) -> (x = 0?=w270:bool)
              n183 = property on="XY-Graph" class="XYGraph (strikt)"("Active Plot"=w266, "Plot.Visible?"=TRUE, "Plot.YScaleIdx"=w264, "Plot.Line Style"=w263) -> ("Plot.Plot Color"=w265:u32)  [unwired: 2 in, 2 out]
              n184 = case shown="False" w270 {
                tunnel: w265 -> [_ w276]
                tunnel: [w273 w275] -> w272
                tunnel: w271 -> [w273 w274]
                frame False {
                }
                frame True {
                  n185 = Insert Into Array(array=w274, new element=w276) -> (w275:u32[])  [unwired: 1 in]
                }
              }
            }
            n186 = for {
              shift-right: [w262] -> _
              shift-left: w249 -> [w259]
              tunnel: w252 -> [w260] mode=indexing
              tunnel: w251 -> [w261]
              tunnel: w250 -> [w258]
              shift-right: [w257] -> _
              shift-left: w249 -> [w256]
              w255 = "\t"
              n187 = Match Pattern(string=w258, regular expression=w255, offset (0)=w256) -> (offset past match=w257:i32)  [unwired: 3 out]
              n188 = Match Pattern(string=w261, regular expression=w255, offset (0)=w259) -> (offset past match=w262:i32)  [unwired: 3 out]
              n189 = property on="Fahrzeugdaten" class="Str"("Text.Selection Start"=w256, "Text.Selection End"=w257, "Text.FontColor"=w260) -> ()  [unwired: 2 in, 2 out]
              n190 = property on="Ergebnis" class="Str"("Text.Selection Start"=w259, "Text.Selection End"=w262, "Text.FontColor"=w260) -> ()  [unwired: 2 in, 2 out]
            }
          }
        }
        n191 = Max & Min(x=w100, y=2) -> (max(x,y)=w101:i32)  [unwired: 1 out]
        n192 = Greater Or Equal?(x=w100, y=14) -> (x >= y?=w132:bool)
        n193 = property on="XY-Graph" class="XYGraph (strikt)"("LegNumRows"=w101) -> ()  [unwired: 2 in, 2 out]
        n194 = case shown="True" w132 {
          frame False {
          }
          frame True {
            n195 = property on="Überlagern" class="Bool. (strikt)"("DisabledEnum"=2) -> ()  [unwired: 2 in, 2 out]
          }
        }
        "Ergebnis" <- w149
        "Fahrzeugdaten" <- w148
      }
      event "Speichern": Value Change {
        n196 = event-data() -> ("OldVal"=w326:bool)  [unwired: 1 in, 5 out]
        n197 = local write "Speichern"(w326) -> ()
        n198 = control-ref of="Datenspeicher"() -> (w325:refnum<vi>)
        n199 = call "savecluster_V0.01.vi"("Datenspeicher 3"=w325) -> ()  [unwired: 2 in]
      }
      event "Stopp": Value Change {
        n200 = event-data() -> ("OldVal"=w327:bool, "NewVal"=w328:bool)  [unwired: 1 in, 4 out]
        n201 = local write "Stopp"(w327) -> ()
      }
      event "Legende": Value Change {
        n202 = event-data() -> ()  [unwired: 1 in, 6 out]
        n203 = local read "XY-Graph"() -> (w332:cluster{dbl[], dbl[]}[])
        n204 = Array Size(array=w332) -> (size(s)=w331:i32)
        n205 = Max & Min(x=w331, y=2) -> (max(x,y)=w329:i32)  [unwired: 1 out]
        n206 = property on="XY-Graph" class="XYGraph (strikt)"("Legend Visible"="Legende", "LegNumRows"=w329) -> ()  [unwired: 2 in, 2 out]
      }
    }
  }
  n207 = property on="Ergebnis" class="Str"("Value"=w12) -> ()  [unwired: 2 in, 2 out]
  n208 = property on="Pmax" class="Str"("Value"=w12) -> ()  [unwired: 2 in, 2 out]
  n209 = property on="Fahrzeugdaten" class="Str"("Value"=w12) -> ()  [unwired: 2 in, 2 out]
  n210 = property on="Datum, Zeit" class="Str"("Value"=w12) -> ()  [unwired: 2 in, 2 out]
  n211 = property on="Fensterbereich" class="Bereich"("Origin"=T3 {"Horizontal"=8, "Vertical"=6}) -> ()  [unwired: 2 in, 2 out]
  n212 = case shown="True" "Berechnen" {
    selector: "Berechnen" -> [_ w337]
    frame False {
    }
    frame True {
      n213 = property on="Berechnen" class="Bool. (strikt)"("Value"=w337, "DisabledEnum"=T4."Enabled" ("Deaktiviert")) -> (error out=w334:errorcluster)  [unwired: 2 in, 1 out]
      n214 = property on="Öffnen" class="Bool. (strikt)"(error in=w334, "Val(Sgnl)"=TRUE ("Wert (signalisierend)")) -> ()  [unwired: 1 in, 2 out]
    }
  }
  n215 = property on="Berechnen" class="Bool. (strikt)"("DisabledEnum"=w4) -> ()  [unwired: 2 in, 2 out]
  n216 = property on="Speichern" class="Bool. (strikt)"("DisabledEnum"=w4) -> ()  [unwired: 2 in, 2 out]
  n217 = property on="Drucken" class="Bool. (strikt)"("DisabledEnum"=w4) -> ()  [unwired: 2 in, 2 out]
  n218 = property on="Fensterbereich" class="Bereich"("Origin"=T3 {"Horizontal"=8, "Vertical"=6}) -> ()  [unwired: 2 in, 2 out]
  n219 = property on="Differenzenquotient" class="DigWert (strikt)"("DisabledEnum"=w2) -> ()  [unwired: 2 in, 2 out]
  n220 = property on="Gl. Mittelwert" class="DigWert (strikt)"("DisabledEnum"=w2) -> ()  [unwired: 2 in, 2 out]
  n221 = property on="Überlagern" class="Bool. (strikt)"("DisabledEnum"=w4) -> ()  [unwired: 2 in, 2 out]
  n222 = Bundle(w8, w8) -> (w6:cluster{dbl[], dbl[]})  [unwired: 1 in]
  n223 = Bundle(w8, w8) -> (w5:cluster{dbl[], dbl[]})  [unwired: 1 in]
  n224 = Build Array(w6, w5) -> (w7:cluster{dbl[], dbl[]}[])
  n225 = property on="XY-Graph" class="XYGraph (strikt)"("Legend Visible"=TRUE, "LegNumRows"=2) -> ()  [unwired: 2 in, 2 out]
  n226 = property on="XY-Graph" class="XYGraph (strikt)"("Value"=w7) -> ()  [unwired: 2 in, 2 out]
